vi "Process_Report_Generator (SubVI).vi"(10 "Process Name":string, 11 "Process Information":string[](array[string])) -> ()   [LabVIEW 2019]
uses:
  <vilib>/Utility/file.llb/Write Delimited Spreadsheet (string).vi
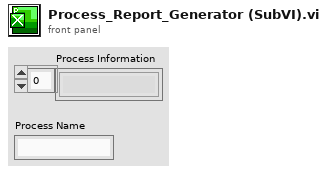
[diagram p1: front panel]
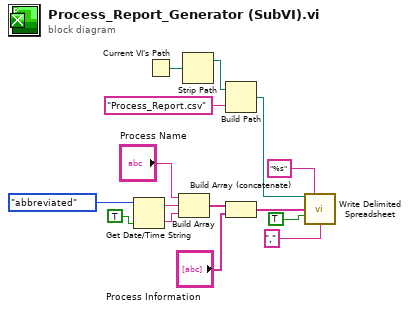
[diagram p0: block diagram]
diagram:
  n1 = Get Date/Time String(date format (0)=enum16{"short", "long", "abbreviated"}."abbreviated", want seconds? (F)=TRUE) -> (date string=w10:string, time string=w11:string)  [unwired: 1 in]
  n2 = Current VI's Path() -> (path=w2:path)
  n3 = Build Array("Process Name", w10, w11) -> (w13:string[])
  n4 = Strip Path(path=w2) -> (stripped path=w1:path)  [unwired: 1 out]
  n5 = Build Path(base path=w1, name or relative path="Process_Report.csv") -> (appended path=w3:path)
  n6 = Build Array (concatenate)(w13, "Process Information") -> (w14:string[])
  n7 = call-poly <vilib>:"Write Delimited Spreadsheet.vi"("file path (dialog if empty)"=w3, "format (%s)"="%s", "1D data"=w14, "append to file? (new file:F)"=TRUE, "delimiter (\\t)"="," ("delimiter (\\t)")) -> ()  [unwired: 9 in, 2 out]
